vi "WPI_Power Get PDP Voltage.vi"(0 "Power Distribution Panel (0)":u8, 11 "error in":errorcluster) -> (6 "voltage (V)":dbl, 15 "error out":errorcluster)   [LabVIEW 2017]
doc: "Returns the battery voltage at the Power Distribution Panel (PDP)."
uses:
  <vilib>/Rock Robotics/WPI/CAN/PDP/WPI_CAN_PDPGlobalOps.ctl
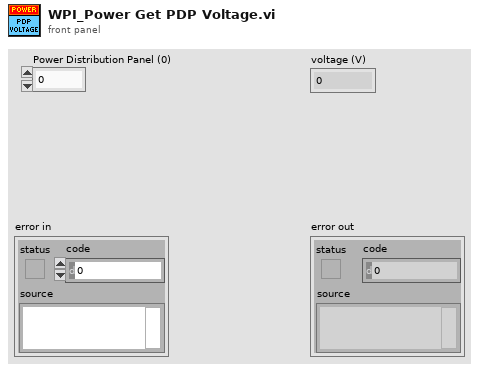
[diagram p1: front panel]
types:
  T1 = typedef "WPI_CAN_PDPGlobalOps.ctl" = enum16{"Write After Receive 0-5", "Write After Receive 6-11", "Write After Receive 12-15", "Write After Receive Energy", "Get All", "Get Commands", "Write Clear Sticky Faults Command", "Write Reset Energy Command", "Write Tare Currents Command", "Write Error", "Write After Receive Faults"}
  T2 = typedef "WPI_CAN_PDPGetAll.ctl" = cluster{"Channel Currents":dbl[], "Battery Voltage":dbl, "Temperature (degrees C)":dbl, "Internal Battery R (Ohms)":dbl, "Energy (J)":dbl, "Power (W)":dbl, "Total Current (A)":dbl, "CAN Error":errorcluster, "Current Faults":bool[], "Battery Voltage Fault":bool, "Temperature Fault":bool, "Hardware Fault":bool}
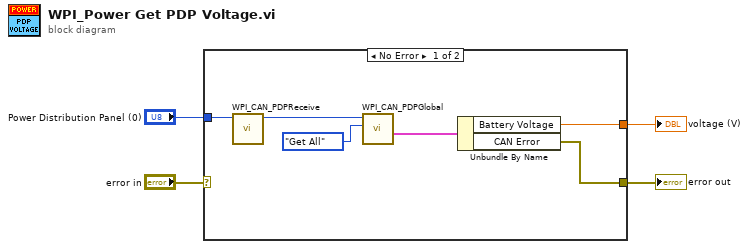
[diagram p0: block diagram]
diagram:
  n1 = case shown="No Error" "error in" {
    selector: "error in" -> [_ w11]
    tunnel: [w5 w11] -> w3
    tunnel: "Power Distribution Panel (0)" -> [w7 _]
    tunnel: [w8 _] -> w1
    frame No Error {
      n2 = call <vilib>:"WPI_CAN_PDPReceive.vi"("Power Distribution Panel (0)"=w7) -> ("Power Distribution Panel Out"=w9:u8)  [unwired: 10 in]
      n3 = call <vilib>:"WPI_CAN_PDPGlobal.vi"("Operation"=WPI_CAN_PDPGlobalOps."Get All", "Power Distribution Panel (0)"=w9) -> ("Get All"=w10:T2)  [unwired: 7 in, 2 out]
      n4 = Unbundle By Name(w10) -> ("Battery Voltage"=w8:dbl, "CAN Error"=w5:errorcluster)
    }
    frame Error {
    }
  }
  "error out" <- w3
  "voltage (V)" <- w1
